vi "radial_array_display.vi"(8 "array":i32[](array[numeric]), 9 "clear (T/F)":bool, 11 "NXT":T1={"Hardware"="NXT", "Flattened String"=""}) -> (3 "NXT 2":T1={"Hardware"="NXT", "Flattened String"=""})   [LabVIEW 2012]
uses:
  <vilib>/NXT/Subs/LVHSConnector.ctl
  <vilib>/NXT/Dual Mode Library/Display/drawNumber.vi
  <vilib>/NXT/Dual Mode Library/Display/drawCircle.vi
  <vilib>/NXT/Dual Mode Library/Display/clearDisplay.vi
  <vilib>/NXT/Dual Mode Library/Display/drawLine.vi
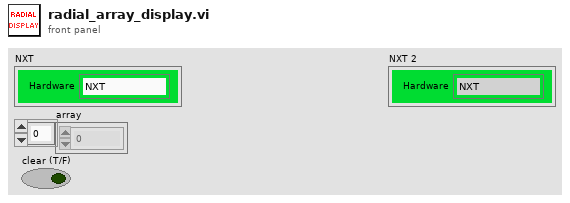
[diagram p1: front panel]
types:
  T1 = typedef "LVHSConnector.ctl" = cluster{"Hardware":string, "Flattened String":string}
  T2 = cluster{"Origin X":i16, "Origin Y":i16, "Radius":u8}
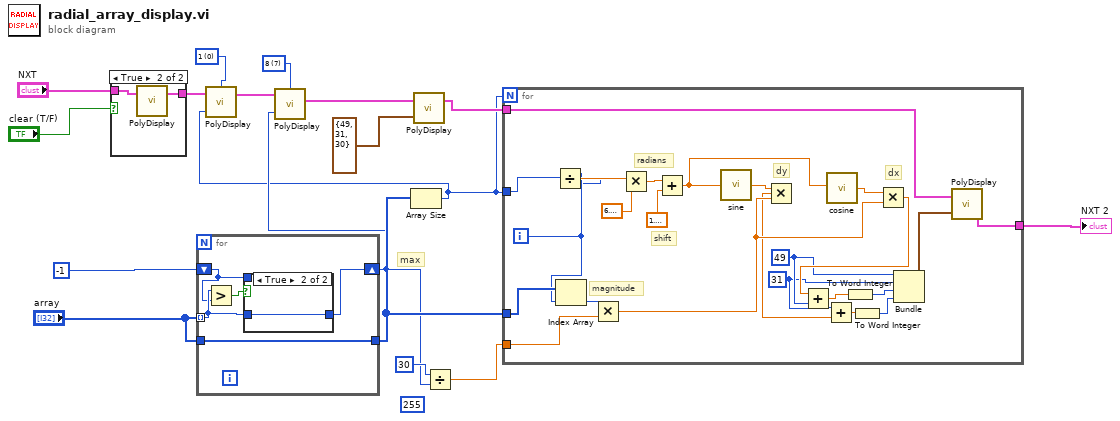
[diagram p0: block diagram]
diagram:
  w5 = i16 0 items=["1", "2", "3", "4", "5", "6", "7", "8"] ("Line")
  w8 = i16 7 items=["1", "2", "3", "4", "5", "6", "7", "8"] ("Line")
  (unwired) i16 255 ("Start X")
  # "max"
  n1 = case shown="True" "clear (T/F)" {
    tunnel: "NXT" -> [w18 w20]
    tunnel: [w18 w19] -> w4
    frame False {
    }
    frame True {
      n2 = call-poly <vilib>:"PolyDisplay.vi"("NXT"=w20) -> ("NXT"=w19:T1)  [unwired: 3 in]
    }
  }
  n3 = for {
    tunnel: "array" -> [w23] mode=indexing
    tunnel: "array" -> [w25]
    tunnel: [w25] -> w13
    shift-right: [w22] -> w7
    shift-left: i16 -1 ("Start X") -> [w21]
    n4 = Greater?(x=w23, y=w21) -> (0:w24:bool)
    n5 = case shown="True" w24 {
      tunnel: w23 -> [_ w27]
      tunnel: [w26 w27] -> w22
      tunnel: w21 -> [w26 _]
      frame False {
      }
      frame True {
      }
    }
  }
  n6 = Array Size(array=w13) -> (size(s)=w3:i32)
  n7 = call-poly <vilib>:"PolyDisplay.vi"("number"=w3, "NXT"=w4, "Line"=w5) -> ("NXT"=w2:T1)  [unwired: 1 in]
  n8 = call-poly <vilib>:"PolyDisplay.vi"("number"=w7, "NXT"=w2, "Line"=w8) -> ("NXT"=w9:T1)  [unwired: 1 in]
  n9 = call-poly <vilib>:"PolyDisplay.vi"("Circle Parameters"=T2 {"Origin X"=49, "Origin Y"=31, "Radius"=30}, "NXT"=w9) -> ("NXT"=w10:T1)  [unwired: 2 in]
  n10 = Divide(x=i16 30 ("Start X"), y=w7) -> (x/y=w17:dbl)
  n11 = for {
    N: w3 -> [_]
    tunnel: [w47] -> w15
    tunnel: w17 -> [w51]
    tunnel: w10 -> [w50]
    tunnel: w13 -> [w49]
    tunnel: w3 -> [w32]
    i -> [w33]
    w41 = i16 49 ("Start X")
    w39 = i16 31 ("Start X")
    # "shift"
    # "dx"
    # "dy"
    # "radians"
    # "magnitude"
    n12 = Divide(x=w33, y=w32) -> (x/y=w46:dbl)
    n13 = Index Array(array=w49, index=w33) -> (element=w48:i32)
    n14 = Multiply(x=w48, y=w51) -> (x*y=w40:dbl)
    n15 = Multiply(x=w46, y=6.283185307179586 ("Pi Multiplied By 2")) -> (x*y=w30:dbl)
    n16 = Add(x=w30, y=1.5707963267948966 ("Pi Divided By 2")) -> (x+y=w29:dbl)
    n17 = call <vilib>:"sine.vi"("x"=w29) -> ("sin(x)"=w44:sgl)
    n18 = Multiply(x=w44, y=w40) -> (x*y=w31:dbl)
    n19 = Add(x=w39, y=w31) -> (x+y=w35:dbl)
    n20 = call <vilib>:"cosine.vi"("x"=w29) -> ("cos(x)"=w43:sgl)
    n21 = To Word Integer(number=w35) -> (16bit integer=w34:i16)
    n22 = Multiply(x=w43, y=w40) -> (x*y=w42:dbl)
    n23 = Add(x=w42, y=w41) -> (x+y=w37:dbl)
    n24 = To Word Integer(number=w37) -> (16bit integer=w36:i16)
    n25 = Bundle("Start X"=w41, "Start X"=w39, w36, w34) -> (w38:cluster{"Start X":i16, "Start X":i16, i16, i16})  [unwired: 1 in]
    n26 = call-poly <vilib>:"PolyDisplay.vi"("Line Parameters"=w38, "NXT"=w50) -> ("NXT"=w47:T1)  [unwired: 2 in]
  }
  "NXT 2" <- w15
